vi "Stop Core.vi"(10 "final error code":i32, 11 "Counter in":refnum<class "Counter.lvclass">) -> (3 "Counter out":refnum<class "Counter.lvclass">)   [LabVIEW 2020, in "Counter.lvlib" / "Counter.lvclass"]
doc: "(<B>Filename</B>: Actor Framework.lvlib:Actor.lvclass:Stop Core.vi)\n\nDefines what the actor does before it stops. Use the <B>final error code</B> input to determine whether the actor shut down in response to an error.\n\nBy default, this method passes the Stop message along to all auto-stop nested actors. A descendant class may override this method to define additional behavior, such as shutting down any processes the actor initiated in its override of the Actor Core method."
uses:
  Counter.lvclass
  <vilib>/ActorFramework/Actor/Actor.lvclass
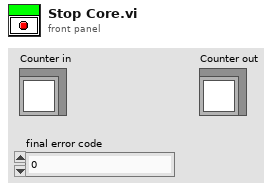
[diagram p1: front panel]
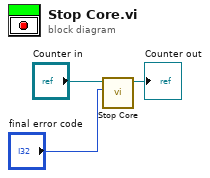
[diagram p0: block diagram]
diagram:
  n1 = call-parent "Stop Core.vi"("final error code"="final error code", "Actor in"="Counter in") -> ("Actor out"=→"Counter out":refnum<class "Counter.lvclass">)  [unwired: 9 in]
